vi "Week 2 Analog Input Samples.vi"() -> ()   [LabVIEW 2022 SP3]
uses:
  <vilib>/DAQmx/read.llb/DAQmx Read (Analog DBL 1Chan 1Samp).vi
  <vilib>/DAQmx/create/channels.llb/DAQmx Create Channel (AI-Voltage-Basic).vi
  <vilib>/DAQmx/configure/timing.llb/DAQmx Timing (Sample Clock).vi
  <vilib>/DAQmx/miscellaneous.llb/DAQmx Fill In Error Info.vi
panel:
  out "Numeric":dbl
  in  "stop":bool
  out "Meter":dbl(knob) scale=0.0..5.0
  out "Waveform Chart":dbl(graph)
  in  "physical channels":tag
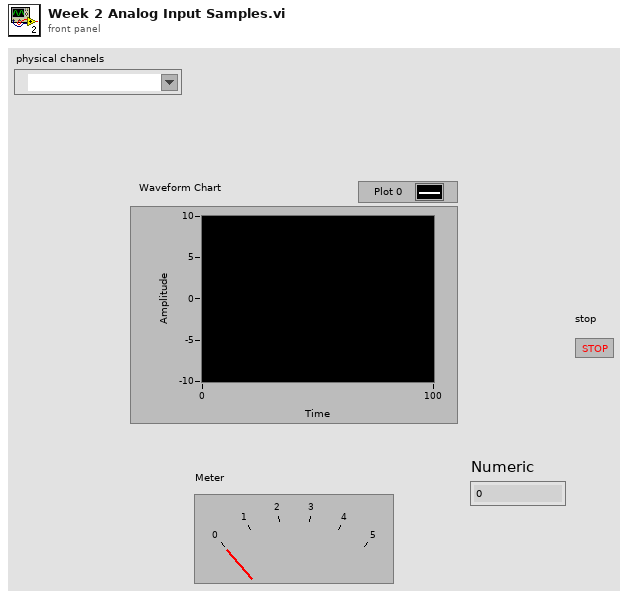
[diagram p1: front panel]
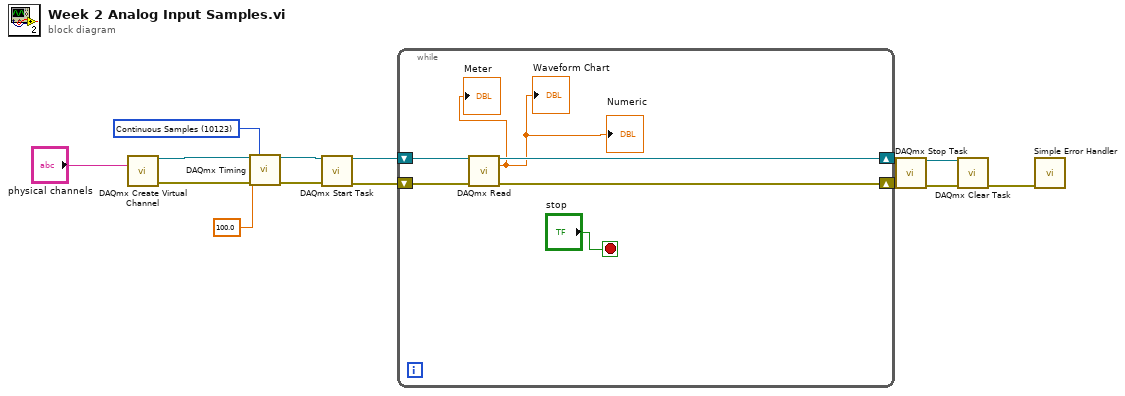
[diagram p0: block diagram]
diagram:
  w2 = 10123 items=["Finite Samples"=10178, "Continuous Samples"=10123, "Hardware Timed Single Point"=12522] ("sample mode")
  n1 = call-poly <vilib>:"DAQmx Create Virtual Channel.vi"("physical channels"="physical channels") -> ("task out"=w6:refnum<k21>, "error out"=w4:errorcluster)  [unwired: 13 in]
  n2 = call-poly <vilib>:"DAQmx Timing.vi"("task/channels in"=w6, "sample mode"=w2, "rate"=100.0, "error in"=w4) -> ("task out"=w5:refnum<k21>, "error out"=w3:errorcluster)  [unwired: 10 in]
  n3 = call <vilib>:"DAQmx Start Task.vi"("task/channels in"=w5, "error in"=w3) -> ("task out"=w14:refnum<k21>, "error out"=w11:errorcluster)  [unwired: 12 in]
  n4 = while {
    shift-right: [w19] -> w13
    shift-left: w14 -> [w20]
    shift-right: [w17] -> w10
    shift-left: w11 -> [w18]
    stop <- "stop" stop-if-true
    n5 = call-poly <vilib>:"DAQmx Read.vi"("task/channels in"=w20, "error in"=w18) -> ("task out"=w19:refnum<k21>, "data"=→"Waveform Chart" →"Meter" →"Numeric":dbl, "error out"=w17:errorcluster)  [unwired: 11 in]
  }
  n6 = call <vilib>:"DAQmx Stop Task.vi"("task/channels in"=w13, "error in"=w10) -> ("task out"=w12:refnum<k21>, "error out"=w9:errorcluster)  [unwired: 12 in]
  n7 = call <vilib>:"DAQmx Clear Task.vi"("task in"=w12, "error in"=w9) -> ("error out"=w7:errorcluster)  [unwired: 13 in]
  n8 = call <vilib>:"Simple Error Handler.vi"("error in (no error)"=w7) -> ()  [unwired: 4 in, 5 out]
